vi "WriteCSV.vi"(7 "Overwrite File if Exists? (F - append suffix)":bool, 8 "error in (no error)":errorcluster, 10 "Data to Write":string[][](array[string]), 11 "file path (empty creates file in temp folder)":path) -> (0 "error out":errorcluster, 3 "actual path":path)   [LabVIEW 2019, in "flashcards.lvlib"]
uses:
  flashcards.lvlib
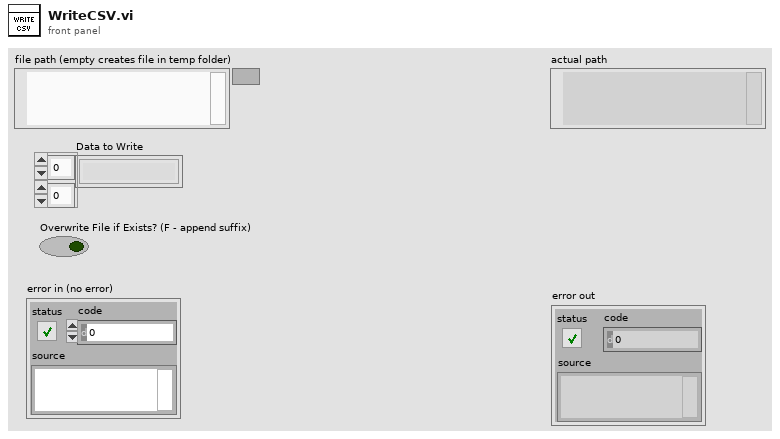
[diagram p1: front panel]
types:
  T1 = enum16{"open", "replace", "create", "open or create", "replace or create", "replace or create with confirmation"}
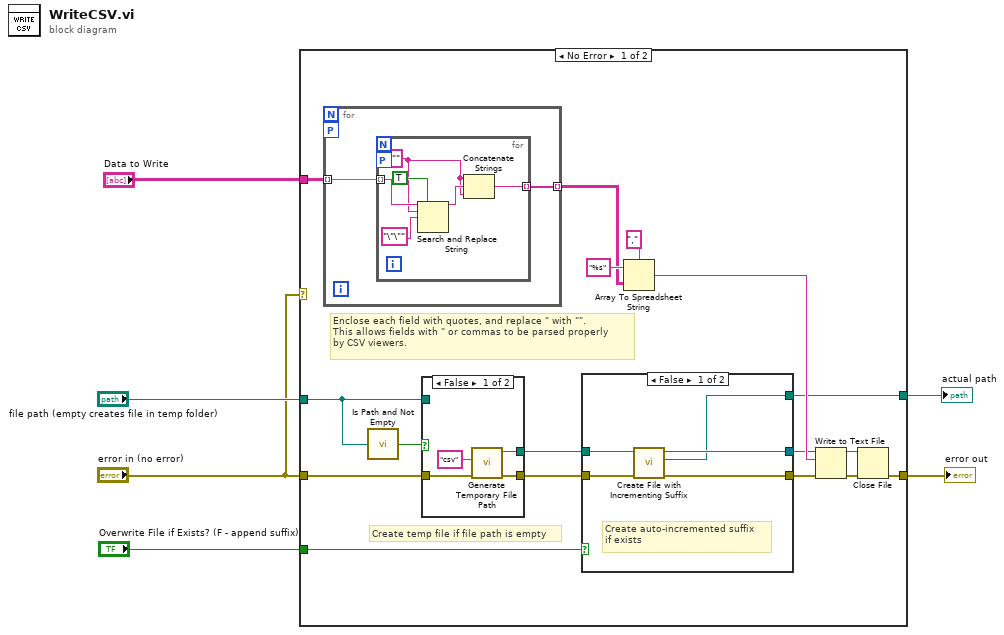
[diagram p0: block diagram]
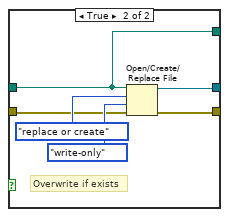
[diagram p2: hidden frame]
diagram:
  n1 = case shown="No Error" "error in (no error)" {
    tunnel: "file path (empty creates file in temp folder)" -> [w11 _]
    tunnel: [w15 _] -> w5
    tunnel: "Data to Write" -> [w14 _]
    tunnel: "error in (no error)" -> [w12 w49]
    tunnel: [w13 w49] -> w3
    tunnel: "Overwrite File if Exists? (F - append suffix)" -> [w7 _]
    frame No Error {
      # "Create temp file if file path is empty"
      # "Enclose each field with quotes, and replace \" with \"\".\nThis allows fields with \" or commas to be parsed properly\nby CSV viewers."
      n2 = for {
        tunnel: w14 -> [w42] mode=indexing
        tunnel: [w41] -> w17 mode=indexing
        workers-P: _ -> [_]
        n3 = for {
          tunnel: w42 -> [w48] mode=indexing
          tunnel: [w43] -> w41 mode=indexing
          workers-P: _ -> [_]
          w44 = "\"" ("search string")
          n4 = Search and Replace String(replace all?=TRUE ("replace all? (F)"), input string=w48, search string=w44, replace string="\"\"" ("replace string (\"\")")) -> (result string=w45:string)  [unwired: 4 in, 3 out]
          n5 = Concatenate Strings(w44, w45, w44) -> (w43:string)
        }
      }
      n6 = call <vilib>:"Is Path and Not Empty.vi"("path"=w11) -> ("Is Path and Not Empty?"=w8:bool)  [unwired: 4 in]
      n7 = case shown="False" w8 {
        tunnel: w12 -> [w37 w40]
        tunnel: [w36 w40] -> w10
        tunnel: [w35 w39] -> w9
        tunnel: w11 -> [_ w39]
        frame False {
          n8 = call <vilib>:"Generate Temporary File Path.vi"("error in (no error)"=w37, "Temporary File Extension (tmp)"="csv") -> ("error out"=w36:errorcluster, "Unique Temporary File Path"=w35:path)  [unwired: 8 in]
        }
        frame True {
        }
      }
      n9 = case shown="False" w7 {
        tunnel: [w28 w30] -> w23
        tunnel: [w27 w31] -> w20
        tunnel: [w26 w29] -> w15
        tunnel: w10 -> [w25 w32]
        tunnel: w9 -> [w24 w29]
        frame False {
          # "Create auto-incremented suffix\nif exists"
          n10 = call <vilib>:"Create File with Incrementing Suffix.vi"("error in (no error)"=w25, "file path"=w24) -> ("error out"=w28:errorcluster, "actual path"=w26:path, "refnum out"=w27:refnum<file>)  [unwired: 7 in]
        }
        frame True {
          # "Overwrite if exists"
          n11 = Open/Create/Replace File(file path (use dialog)=w29, error in=w32, operation (0:open)=T1."replace or create", access (0:read/write)=enum16{"read/write", "read-only", "write-only"}."write-only") -> (refnum out=w31:refnum<file>, error out=w30:errorcluster)  [unwired: 2 in, 1 out]
        }
      }
      n12 = Array To Spreadsheet String(delimiter (Tab)=",", array=w17, 3:"%s" ("format string")) -> (spreadsheet string=w21:string)
      n13 = Write to Text File(file (use dialog)=w20, text=w21, error in=w23) -> (refnum out=w18:refnum<file>, error out=w19:errorcluster)  [unwired: 1 in, 1 out]
      n14 = Close File(refnum=w18, error in=w19) -> (error out=w13:errorcluster)  [unwired: 1 out]
    }
    frame Error {
    }
  }
  "actual path" <- w5
  "error out" <- w3
